vi "Close Color Processors.vi"(8 "error in (no error)":errorcluster, 11 "Color Processor References":T1) -> (0 "error out":errorcluster)   [LabVIEW 2022 SP3]
uses:
  Color/Color Processor References.ctl
  I:/.shortcut-targets-by-id/1riZacJd_1_jmKfGgrjDuP7KcecvMS3i2/Xiao research group/Programs/XYZRecorrection/Scientific Camera Interfaces/SDK/DotNet Toolkit/dlls/Managed_64_lib/Thorlabs.TSI.Demosaicker.dll
  SDK/DotNet Toolkit/dlls/Managed_64_lib/Thorlabs.TSI.Demosaicker.dll
  I:/.shortcut-targets-by-id/1riZacJd_1_jmKfGgrjDuP7KcecvMS3i2/Xiao research group/Programs/XYZRecorrection/Scientific Camera Interfaces/SDK/DotNet Toolkit/dlls/Managed_64_lib/Thorlabs.TSI.ColorProcessor.dll
  SDK/DotNet Toolkit/dlls/Managed_64_lib/Thorlabs.TSI.ColorProcessor.dll
  I:/.shortcut-targets-by-id/1riZacJd_1_jmKfGgrjDuP7KcecvMS3i2/Xiao research group/Programs/XYZRecorrection/Scientific Camera Interfaces/SDK/DotNet Toolkit/dlls/Managed_64_lib/Thorlabs.TSI.ColorInterfaces.dll
  SDK/DotNet Toolkit/dlls/Managed_64_lib/Thorlabs.TSI.ColorInterfaces.dll
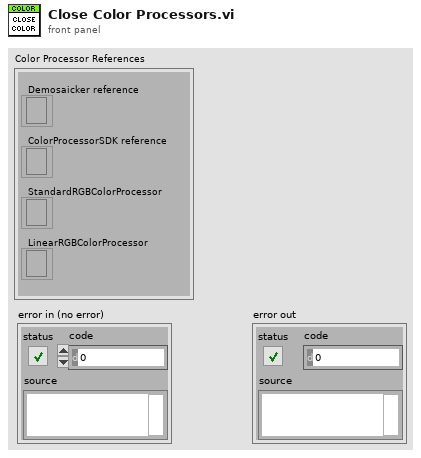
[diagram p1: front panel]
types:
  T1 = typedef "Color Processor References.ctl" = cluster{"Demosaicker reference":refnum<k24>, "ColorProcessorSDK reference":refnum<k24>, "StandardRGBColorProcessor":refnum<k24>, "LinearRGBColorProcessor":refnum<k24>}
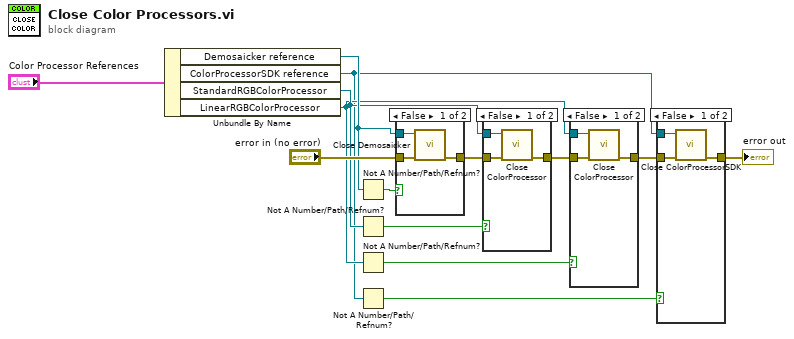
[diagram p0: block diagram]
diagram:
  n1 = Unbundle By Name("Color Processor References") -> ("Demosaicker reference"=w11:refnum<k24>, "ColorProcessorSDK reference"=w3:refnum<k24>, "StandardRGBColorProcessor"=w8:refnum<k24>, "LinearRGBColorProcessor"=w7:refnum<k24>)
  n2 = Not A Number/Path/Refnum?(number/path/refnum=w11) -> (NaN/Path/Refnum?=w13:bool)
  n3 = Not A Number/Path/Refnum?(number/path/refnum=w8) -> (NaN/Path/Refnum?=w9:bool)
  n4 = Not A Number/Path/Refnum?(number/path/refnum=w7) -> (NaN/Path/Refnum?=w6:bool)
  n5 = Not A Number/Path/Refnum?(number/path/refnum=w3) -> (NaN/Path/Refnum?=w4:bool)
  n6 = case shown="False" w13 {
    tunnel: "error in (no error)" -> [w17 w18]
    tunnel: w11 -> [w16 _]
    tunnel: [w15 w18] -> w10
    frame False {
      n7 = call "Close Demosaicker.vi"("error in (no error)"=w17, "Thorlabs.TSI.Demosaicker.Demosaicker"=w16) -> ("error out"=w15:errorcluster)  [unwired: 9 in]
    }
    frame True {
    }
  }
  n8 = case shown="False" w9 {
    tunnel: w10 -> [w21 w22]
    tunnel: w8 -> [w19 _]
    tunnel: [w20 w22] -> w5
    frame False {
      n9 = call "Close ColorProcessor.vi"("error in (no error)"=w21, "Thorlabs.TSI.ColorInterfaces.IColorProcessor"=w19) -> ("error out"=w20:errorcluster)  [unwired: 9 in]
    }
    frame True {
    }
  }
  n10 = case shown="False" w6 {
    tunnel: w5 -> [w25 w26]
    tunnel: w7 -> [w24 _]
    tunnel: [w23 w26] -> w2
    frame False {
      n11 = call "Close ColorProcessor.vi"("error in (no error)"=w25, "Thorlabs.TSI.ColorInterfaces.IColorProcessor"=w24) -> ("error out"=w23:errorcluster)  [unwired: 9 in]
    }
    frame True {
    }
  }
  n12 = case shown="False" w4 {
    tunnel: w2 -> [w29 w30]
    tunnel: w3 -> [w28 _]
    tunnel: [w27 w30] -> w1
    frame False {
      n13 = call "Close ColorProcessorSDK.vi"("error in (no error)"=w29, "Thorlabs.TSI.ColorProcessor.ColorProcessorSDK"=w28) -> ("error out"=w27:errorcluster)  [unwired: 9 in]
    }
    frame True {
    }
  }
  "error out" <- w1
